vi "Move to pos2go.vi"(0 "Current coordinates":cluster{"X":dbl, "Y":dbl, "Z":dbl}, 1 "DelX":T3={"Go x"=FALSE, "Back x"=FALSE, "Go y"=FALSE, "Back y"=FALSE, "Go z"=FALSE, "Back z"=FALSE, "dX (um)"=1000.0, "dY (um)"=0.0, "dZ (um)"=0.0} {"dX (um)" step=1.0}, 2 "X0":T1={"X (um)"=1000.0, "X 2"=FALSE, "Y (um)"=0.0, "Y 2"=FALSE, "Z (um)"=0.0, "Z 2"=FALSE} {"Y (um)" min=0.0; "X (um)" min=0.0}, 3 "Scaling":cluster{"X":u16, "Y":u16, "Z":u16} {"Z" items=["X", "Z", "None"]; "Y" items=["X", "Z", "None"]; "X" items=["X", "Z", "None"]}, 4 "Mode":u16(ring) items=["GoTo", "Jog"]) -> (5 "Position":T2={"X"=FALSE, "Target X (um)"=1000.0, "Current X (um)"=1000.0, "Scaling X"=0, "Y"=FALSE, "Target Y (um)"=0.0, "Current Y (um)"=0.0, "Scaling Y"=0, "Z"=FALSE, "Target Z (um)"=0.0, "Current Z (um)"=0.0, "Scaling Z"=0} {"Current X (um)" step=1.0; "Scaling Z" items=["X", "Z", "None"]; "Scaling Y" items=["X", "Z", "None"]; "Scaling X" items=["X", "Z", "None"]; "Target X (um)" step=1.0}, 6 "DelX 2":T3={"Go x"=FALSE, "Back x"=FALSE, "Go y"=FALSE, "Back y"=FALSE, "Go z"=FALSE, "Back z"=FALSE, "dX (um)"=1000.0, "dY (um)"=0.0, "dZ (um)"=0.0} {"dX (um)" step=1.0})   [LabVIEW 2018]
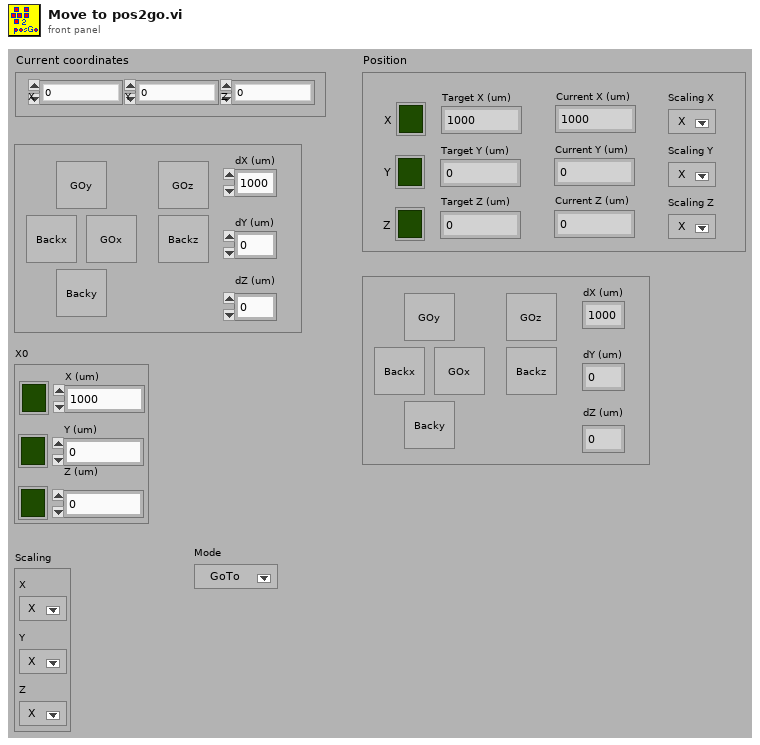
[diagram p1: front panel]
types:
  T1 = cluster{"X (um)":dbl, "X 2":bool, "Y (um)":dbl, "Y 2":bool, "Z (um)":dbl, "Z 2":bool}
  T2 = cluster{"X":bool, "Target X (um)":dbl, "Current X (um)":dbl, "Scaling X":u16, "Y":bool, "Target Y (um)":dbl, "Current Y (um)":dbl, "Scaling Y":u16, "Z":bool, "Target Z (um)":dbl, "Current Z (um)":dbl, "Scaling Z":u16}
  T3 = cluster{"Go x":bool, "Back x":bool, "Go y":bool, "Back y":bool, "Go z":bool, "Back z":bool, "dX (um)":dbl, "dY (um)":dbl, "dZ (um)":dbl}
  T4 = cluster{"Back x":bool, "X":dbl, "dX (um)":dbl, "X":u16, "Back y":bool, "Y":dbl, "dY (um)":dbl, "Y":u16, "Back z":bool, "Z":dbl, "dZ (um)":dbl, "Z":u16}
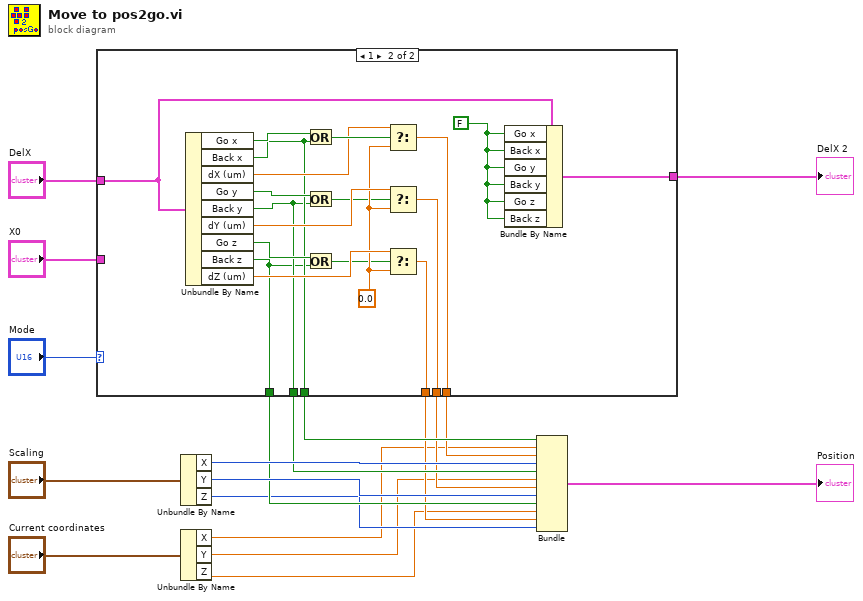
[diagram p0: block diagram]
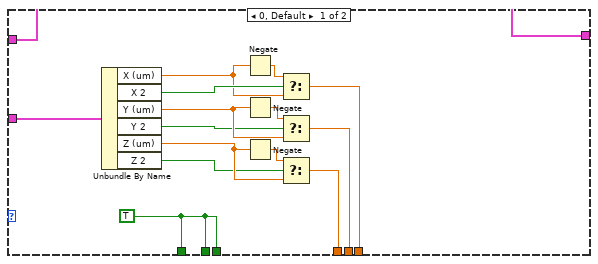
[diagram p2: hidden frame]
diagram:
  n1 = case shown="1" "Mode" {
    tunnel: "DelX" -> [w33 w53]
    tunnel: [w33 w51] -> w17
    tunnel: [w34 w42] -> w16
    tunnel: [w21 w41] -> w15
    tunnel: [w34 w40] -> w13
    tunnel: [w22 w39] -> w12
    tunnel: [w34 w38] -> w10
    tunnel: [w23 w37] -> w9
    tunnel: "X0" -> [w20 _]
    frame 0, Default {
      w34 = TRUE
      n2 = Unbundle By Name(w20) -> ("X (um)"=w30:dbl, "X 2"=w31:bool, "Y (um)"=w28:dbl, "Y 2"=w27:bool, "Z (um)"=w25:dbl, "Z 2"=w24:bool)
      n3 = Negate(x=w30) -> (-x=w32:dbl)
      n4 = Negate(x=w28) -> (-x=w29:dbl)
      n5 = Negate(x=w25) -> (-x=w26:dbl)
      n6 = Select(t=w32, s=w31, f=w30) -> (s? t:f=w21:dbl)
      n7 = Select(t=w29, s=w27, f=w28) -> (s? t:f=w22:dbl)
      n8 = Select(t=w26, s=w24, f=w25) -> (s? t:f=w23:dbl)
    }
    frame 1 {
      w43 = 0.0
      w52 = FALSE ("Go x")
      n9 = Unbundle By Name(w53) -> ("Go x"=w50:bool, "Back x"=w42:bool, "dX (um)"=w46:dbl, "Go y"=w49:bool, "Back y"=w40:bool, "dY (um)"=w45:dbl, "Go z"=w48:bool, "Back z"=w38:bool, "dZ (um)"=w44:dbl)
      n10 = Or(x=w50, y=w42) -> (x .or. y?=w47:bool)
      n11 = Or(x=w49, y=w40) -> (x .or. y?=w36:bool)
      n12 = Or(x=w48, y=w38) -> (x .or. y?=w35:bool)
      n13 = Select(t=w46, s=w47, f=w43) -> (s? t:f=w41:dbl)
      n14 = Select(t=w45, s=w36, f=w43) -> (s? t:f=w39:dbl)
      n15 = Select(t=w44, s=w35, f=w43) -> (s? t:f=w37:dbl)
      n16 = Bundle By Name(cluster=w53, "Go x"=w52, "Back x"=w52, "Go y"=w52, "Back y"=w52, "Go z"=w52, "Back z"=w52) -> (w51:T3)
    }
  }
  "DelX 2" <- w17
  n17 = Unbundle By Name("Scaling") -> ("X"=w14:u16, "Y"=w11:u16, "Z"=w8:u16)
  n18 = Unbundle By Name("Current coordinates") -> ("X"=w6:dbl, "Y"=w5:dbl, "Z"=w4:dbl)
  n19 = Bundle("Back x"=w16, "X"=w6, "dX (um)"=w15, "X"=w14, "Back y"=w13, "Y"=w5, "dY (um)"=w12, "Y"=w11, "Back z"=w10, "Z"=w4, "dZ (um)"=w9, "Z"=w8) -> (→"Position":T4)  [unwired: 1 in]
